vi "save.vi"(0 "存盘数据":string, 1 "时间":string, 2 "数据（使用对话框）":path, 3 "次数（使用对话框）":path) -> ()   [LabVIEW 2018]
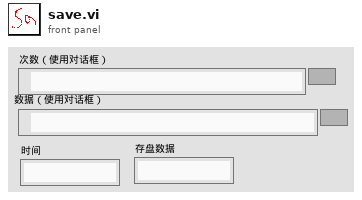
[diagram p1: front panel]
types:
  T1 = enum16{"open", "replace", "create", "open or create", "replace or create", "replace or create with confirmation"}
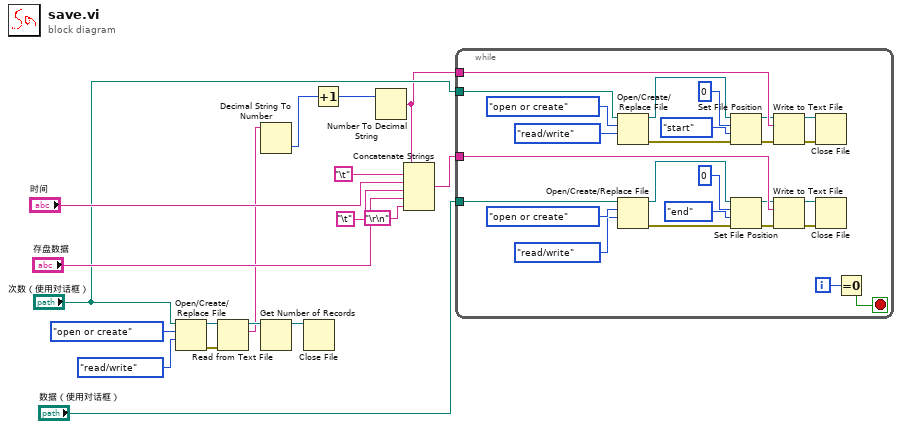
[diagram p0: block diagram]
diagram:
  n1 = Open/Create/Replace File(file path (use dialog)="次数（使用对话框）", operation (0:open)=T1."open or create" ("操作(0:open)"), access (0:read/write)=enum16{"read/write", "read-only", "write-only"}."read/write" ("权限(0:read/write)")) -> (refnum out=w16:refnum<file>, error out=w15:errorcluster)  [unwired: 3 in, 1 out]
  n2 = Read from Text File(file (use dialog)=w16, error in=w15) -> (refnum out=w14:refnum<file>, text=w4:string)  [unwired: 2 in, 2 out]
  n3 = Decimal String To Number(string=w4) -> (number=w3:i32)  [unwired: 2 in, 1 out]
  n4 = Get Number of Records(7:w14) -> (3:w13:refnum<file>)  [unwired: 1 in, 2 out]
  n5 = Close File(refnum=w13) -> ()  [unwired: 1 in, 2 out]
  n6 = Increment(x=w3) -> (x+1=w6:i32)
  n7 = Number To Decimal String(number=w6) -> (decimal integer string=w2:string)  [unwired: 1 in]
  n8 = Concatenate Strings(w2, "\t", "时间", "\t", "存盘数据", "\r\n") -> (w8:string)
  n9 = while {
    tunnel: w8 -> [w41]
    tunnel: "数据（使用对话框）" -> [w33]
    tunnel: w2 -> [w30]
    tunnel: "次数（使用对话框）" -> [w29]
    i -> [w43]
    stop <- w42 stop-if-true
    n10 = Open/Create/Replace File(file path (use dialog)=w29, operation (0:open)=T1."open or create" ("操作(0:open)"), access (0:read/write)=enum16{"read/write", "read-only", "write-only"}."read/write" ("权限(0:read/write)")) -> (refnum out=w26:refnum<file>, error out=w25:errorcluster)  [unwired: 3 in, 1 out]
    n11 = Open/Create/Replace File(file path (use dialog)=w33, operation (0:open)=T1."open or create" ("操作(0:open)"), access (0:read/write)=enum16{"read/write", "read-only", "write-only"}."read/write" ("权限(0:read/write)")) -> (refnum out=w39:refnum<file>, error out=w38:errorcluster)  [unwired: 3 in, 1 out]
    n12 = Set File Position(offset (in bytes) (0)=i64 0 ("偏移量（字节）（0）"), refnum=w26, from (0:start)=enum16{"start", "end", "current"}."start" ("自（0:起始）"), error in=w25) -> (refnum out=w23:refnum<file>, error out=w22:errorcluster)
    n13 = Set File Position(offset (in bytes) (0)=i64 0 ("偏移量（字节）（0）"), refnum=w39, from (0:start)=enum16{"start", "end", "current"}."end" ("自（0:起始）"), error in=w38) -> (refnum out=w37:refnum<file>, error out=w36:errorcluster)
    n14 = Write to Text File(file (use dialog)=w23, text=w30, error in=w22) -> (refnum out=w21:refnum<file>, error out=w20:errorcluster)  [unwired: 1 in, 1 out]
    n15 = Write to Text File(file (use dialog)=w37, text=w41, error in=w36) -> (refnum out=w32:refnum<file>, error out=w31:errorcluster)  [unwired: 1 in, 1 out]
    n16 = Close File(refnum=w21, error in=w20) -> ()  [unwired: 2 out]
    n17 = Close File(refnum=w32, error in=w31) -> ()  [unwired: 2 out]
    n18 = Equal To 0?(x=w43) -> (x = 0?=w42:bool)
  }
